vi "Read Decorations.vi"(9 "Pane in":refnum<class "Pane.lvclass">) -> (3 "Pane out":refnum<class "Pane.lvclass">, 4 "Decorations":refnum<class "Decoration.lvclass">[](array[class]))   [LabVIEW 2014, in "Pane.lvclass"]
uses:
  Pane.lvclass
  Decoration/Decoration.lvclass
  Pane.lvclass/Pane.ctl
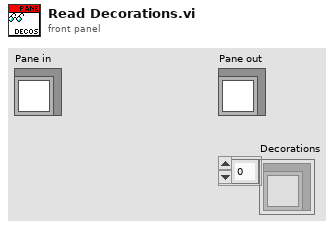
[diagram p1: front panel]
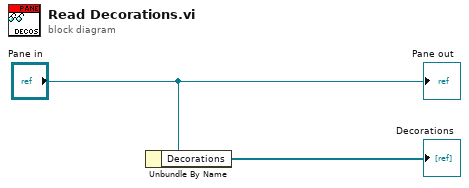
[diagram p0: block diagram]
diagram:
  n1 = Unbundle By Name("Pane in") -> ("Decorations"=→"Decorations":refnum<class "Decoration.lvclass">[])
  "Pane out" <- "Pane in"
